vi "Test_CommonTypes_NamesOK.vi"(8 "error in (no error)":errorcluster, 11 "TestCase in":refnum<class "TestVariantExtensions.lvclass">) -> (0 "error out":errorcluster, 3 "TestCase out":refnum<class "TestVariantExtensions.lvclass">)   [LabVIEW 2015, in "TestVariantExtensions.lvclass"]
uses:
  TestVariantExtensions.lvclass
  <vilib>/addons/_JKI Toolkits/VI Tester/TestCase.llb/TestCase.lvclass
  VariantExtensions.lvlib
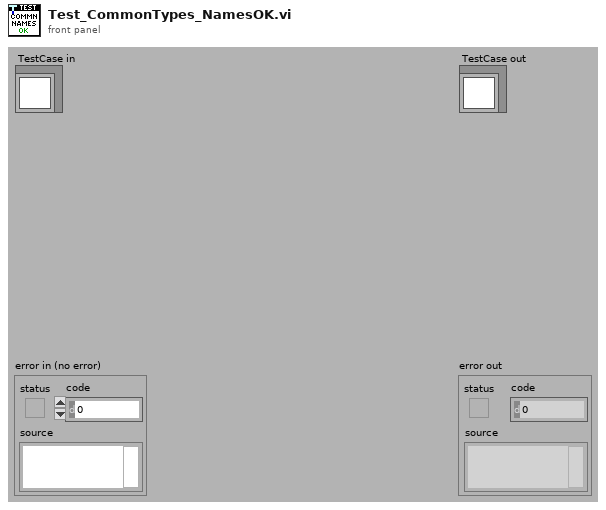
[diagram p1: front panel]
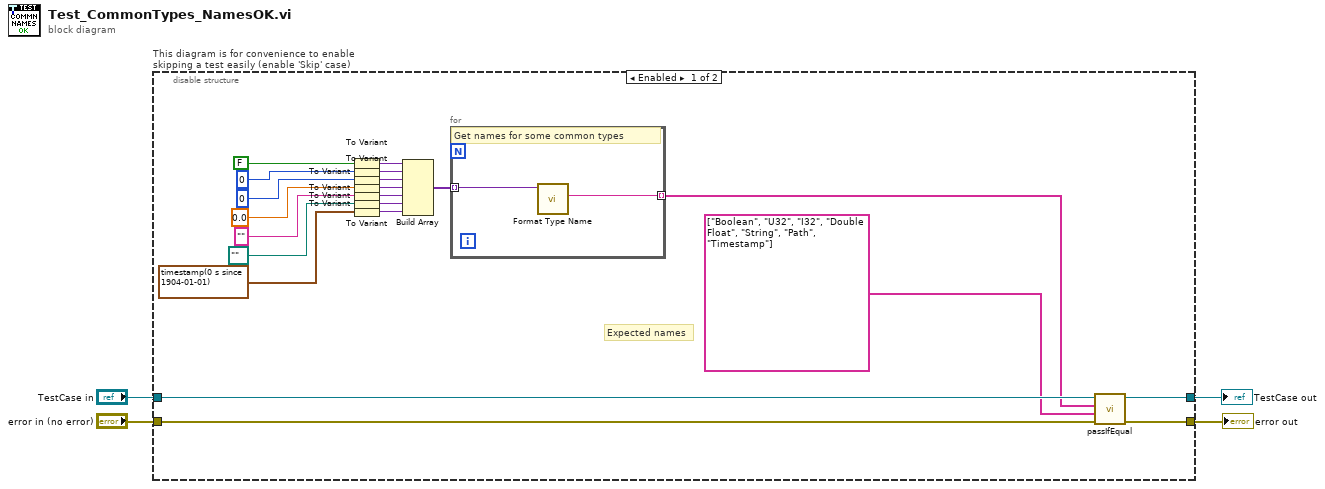
[diagram p0: block diagram]
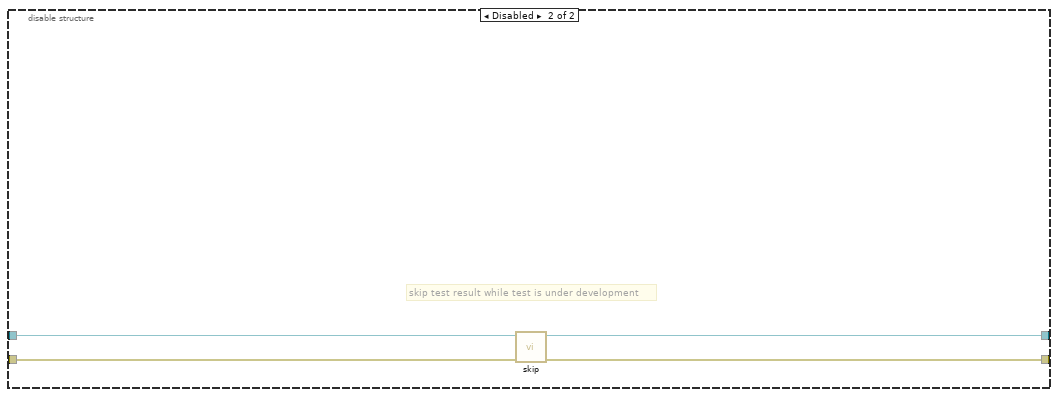
[diagram p2: hidden frame]
diagram:
  n1 = disable-structure "This diagram is for convenience to enable skipping a test easily (enable 'Skip' case)" shown="Enabled" {
    disable-tunnel: "TestCase in" -> [w25 w31]
    disable-tunnel: [w24 w29] -> w1
    disable-tunnel: [w23 w30] -> w3
    disable-tunnel: "error in (no error)" -> [w22 w28]
    frame Enabled {
      # "Expected names"
      n2 = To Variant(anything=FALSE) -> (Variant=w5:variant)
      n3 = To Variant(anything=u32 0) -> (Variant=w21:variant)
      n4 = To Variant(anything=0) -> (Variant=w20:variant)
      n5 = To Variant(anything=0.0) -> (Variant=w19:variant)
      n6 = To Variant(anything="") -> (Variant=w18:variant)
      n7 = To Variant(anything=path "") -> (Variant=w17:variant)
      n8 = To Variant(anything=timestamp(0 s since 1904-01-01)) -> (Variant=w16:variant)
      n9 = Build Array(w5, w21, w20, w19, w18, w17, w16) -> (w9:variant[])
      n10 = for {
        tunnel: [w27] -> w8 mode=indexing
        tunnel: w9 -> [w26] mode=indexing
        # "Get names for some common types"
        n11 = call "Format Type Name.vi"("Data Type"=w26) -> ("Type Name"=w27:string)  [unwired: 9 in, 1 out]
      }
      n12 = call-dynamic "passIfEqual.vi"("error in (no error)"=w22, "y"=string[] ["Boolean", "U32", "I32", "Double Float", "String", "Path", "Timestamp"], "x"=w8, "TestCase in"=w25) -> ("error out"=w23:errorcluster, "TestCase out"=w24:refnum<class "TestVariantExtensions.lvclass">)  [unwired: 6 in]
    }
    frame Disabled {
      # "skip test result while test is under development"
      n13 = call <vilib>:"skip.vi"("error in (no error)"=w28, "TestCase in"=w31) -> ("error out"=w30:errorcluster, "TestCase out"=w29:refnum<class "TestVariantExtensions.lvclass">)  [unwired: 8 in]
    }
  }
  "error out" <- w3
  "TestCase out" <- w1
